vi "Initialize Attributes.vi"(8 "error in (no error)":errorcluster, 10 "Attribute Data":variant, 11 "BNT_DSCXtGraph in":refnum<class "BNT_DSCXtGraph.lvclass">) -> (0 "error out":errorcluster, 2 "Found?":bool, 3 "BNT_DSCXtGraph out":refnum<class "BNT_DSCXtGraph.lvclass">)   [LabVIEW 2015, in "BNT_DSCXtGraph.lvlib" / "BNT_DSCXtGraph.lvclass"]
doc: "Initialize object attribute.\n\nUnique resources should be allocated elsewhere!"
uses:
  BNT_DSCXtGraph.lvclass
  BNT_DSCXtGraph.lvclass/BNT_DSCXtGraph.ctl
  CSPP_Core/Actors/CS++GUIActor/CS++GUIActor.lvclass
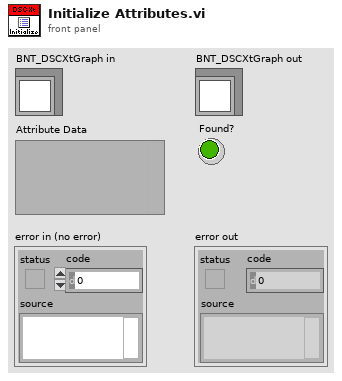
[diagram p1: front panel]
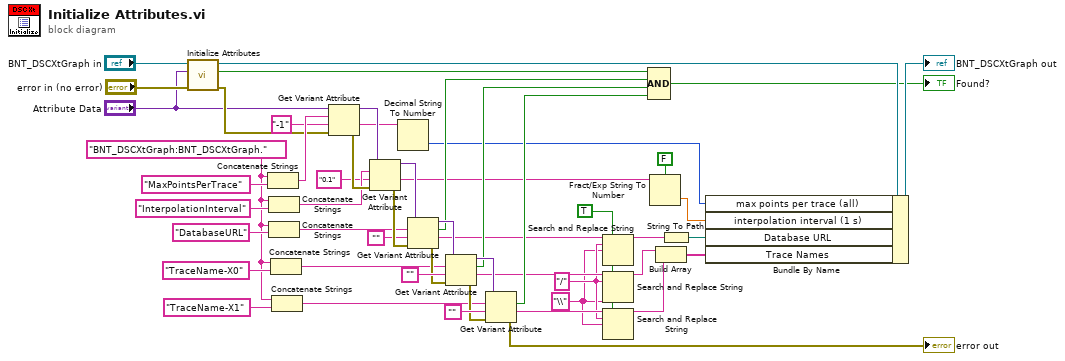
[diagram p0: block diagram]
diagram:
  w9 = TRUE ("replace all? (F)")
  w7 = "\\" ("replace string (\"\")")
  w8 = "/" ("search string")
  w41 = "BNT_DSCXtGraph:BNT_DSCXtGraph."
  n1 = call-parent "Initialize Attributes.vi"("error in (no error)"="error in (no error)", "Attribute Data"="Attribute Data", "CS++GUIActor in"="BNT_DSCXtGraph in") -> ("error out"=w47:errorcluster, "Found?"=w48:bool, "CS++GUIActor out"=w16:refnum<class "BNT_DSCXtGraph.lvclass">)  [unwired: 6 in]
  n2 = Concatenate Strings(w41, "MaxPointsPerTrace" ("string")) -> (w52:string)
  n3 = Concatenate Strings(w41, "InterpolationInterval" ("string")) -> (w49:string)
  n4 = Concatenate Strings(w41, "DatabaseURL" ("string")) -> (w36:string)
  n5 = Concatenate Strings(w41, "TraceName-X0" ("string")) -> (w31:string)
  n6 = Concatenate Strings(w41, "TraceName-X1" ("string")) -> (w27:string)
  n7 = Get Variant Attribute(Variant="Attribute Data", name=w52, default value (empty Variant)="-1" ("string"), error in=w47) -> (duplicate Variant=w51:variant, value=w21:string, error out=w50:errorcluster)  [unwired: 1 out]
  n8 = Get Variant Attribute(Variant=w51, name=w49, default value (empty Variant)="0.1" ("string"), error in=w50) -> (duplicate Variant=w38:variant, value=w19:string, error out=w37:errorcluster)  [unwired: 1 out]
  n9 = Decimal String To Number(string=w21) -> (number=w20:i32)  [unwired: 2 in, 1 out]
  n10 = Get Variant Attribute(Variant=w38, name=w36, default value (empty Variant)="", error in=w37) -> (duplicate Variant=w33:variant, found=w26:bool, value=w10:string, error out=w32:errorcluster)
  n11 = Get Variant Attribute(Variant=w33, name=w31, default value (empty Variant)="", error in=w32) -> (duplicate Variant=w28:variant, found=w25:bool, value=w15:string, error out=w29:errorcluster)
  n12 = Get Variant Attribute(Variant=w28, name=w27, default value (empty Variant)="", error in=w29) -> (found=w24:bool, value=w13:string, error out=→"error out":errorcluster)  [unwired: 1 out]
  n13 = Search and Replace String(replace all?=w9, input string=w10, search string=w8, replace string=w7) -> (result string=w11:string)  [unwired: 4 in, 3 out]
  n14 = Search and Replace String(replace all?=w9, input string=w15, search string=w8, replace string=w7) -> (result string=w14:string)  [unwired: 4 in, 3 out]
  n15 = Search and Replace String(replace all?=w9, input string=w13, search string=w8, replace string=w7) -> (result string=w12:string)  [unwired: 4 in, 3 out]
  n16 = Compound Arithmetic op=AND(w48, w26, w25, w24) -> (→"Found?":bool)
  n17 = Fract/Exp String To Number(use system decimal point (T)=FALSE, string=w19) -> (number=w18:dbl)  [unwired: 2 in, 1 out]
  n18 = Build Array(w14, w12) -> (w22:string[])
  n19 = String To Path(string=w11) -> (path=w23:path)
  n20 = Bundle By Name(cluster=w16, "max points per trace (all)"=w20, "interpolation interval (1 s)"=w18, "Database URL"=w23, "Trace Names"=w22) -> (→"BNT_DSCXtGraph out":refnum<class "BNT_DSCXtGraph.lvclass">)
